vi "GameInit.vi"(8 "error in":errorcluster) -> (0 "error out":errorcluster, 3 "InitCluster":T1)   [LabVIEW 2022 SP3]
uses:
  InitCluster.ctl
  CharacterCluster.ctl
  <vilib>/picture/picture.llb/imagedata.ctl
  ShotInitCluster.ctl
  <vilib>/Utility/miscctls.llb/LVPositionTypeDef.ctl
  <vilib>/Utility/miscctls.llb/LVBoundsTypeDef.ctl
  ShotCluster.ctl
  move_dir_ud.ctl
  SelectPictureToRead.ctl
  ShipShootEnum.ctl
  <vilib>/Utility/config.llb/Read Key (U32).vi
  <vilib>/Utility/config.llb/Read Key (I32).vi
  <vilib>/Utility/config.llb/NI_LVConfig.lvlib
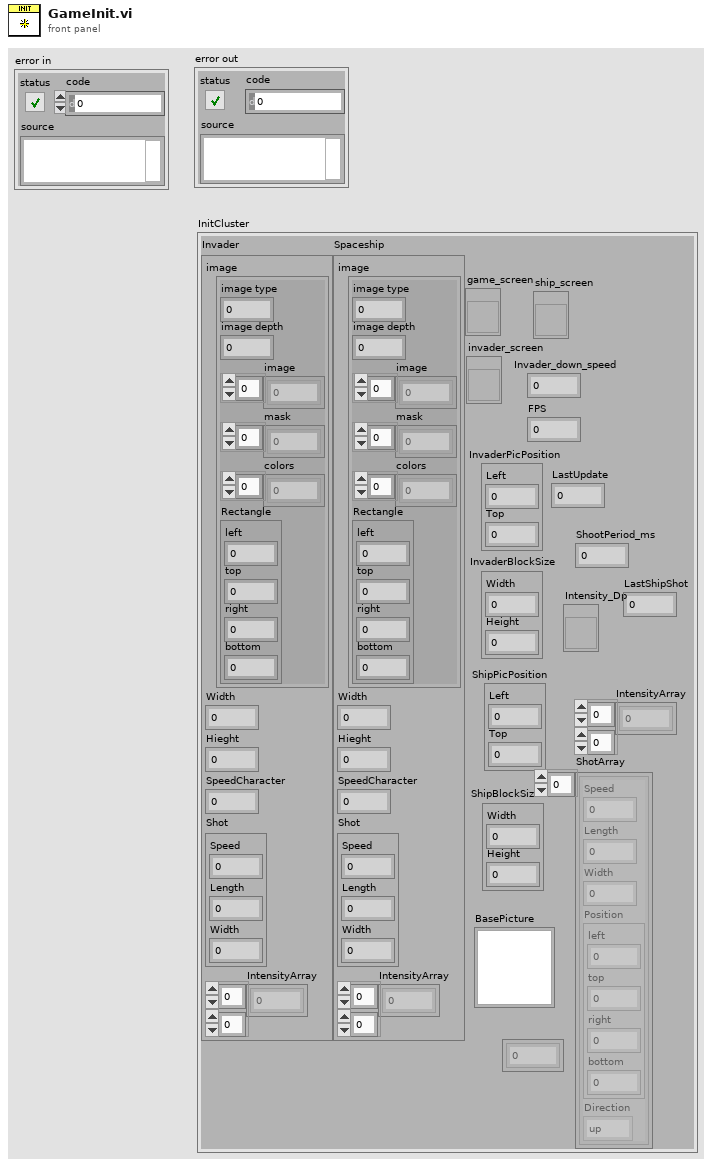
[diagram p1: front panel]
types:
  T1 = typedef "InitCluster.ctl" = cluster{"Invader":T2, "Spaceship":T2, "game_screen":refnum<vi>, "BasePicture":picture, "invader_screen":refnum<vi>, "InvaderPicPosition":T5, "Invader_down_speed":i16, "FPS":u16, "InvaderBlockSize":T6, "ship_screen":refnum<vi>, "ShipBlockSize":T6, "ShipPicPosition":T5, "LastUpdate":u32, "Intensity_Dp":refnum<vi>, "IntensityArray":u8[][], "ShotArray":T7[], "InvaderShotTimeArray":u32[], "ShootPeriod_ms":i32, "LastShipShot":u32}
  T2 = typedef "CharacterCluster.ctl" = cluster{"image":T3, "Width":u32, "Hieght":u32, "SpeedCharacter":u32, "Shot":T4, "IntensityArray":u8[][]}
  T3 = typedef "imagedata.ctl" = cluster{"image type":i32, "image depth":i32, "image":u8[], "mask":u8[], "colors":u32[], "Rectangle":cluster{"left":i16, "top":i16, "right":i16, "bottom":i16}}
  T4 = typedef "ShotInitCluster.ctl" = cluster{"Speed":u32, "Length":u32, "Width":u32}
  T5 = typedef "LVPositionTypeDef.ctl" = cluster{"Left":i32, "Top":i32}
  T6 = typedef "LVBoundsTypeDef.ctl" = cluster{"Width":u32, "Height":u32}
  T7 = typedef "ShotCluster.ctl" = cluster{"Speed":u32, "Length":u32, "Width":u32, "Position":cluster{"left":i16, "top":i16, "right":i16, "bottom":i16}, "Direction":T8}
  T8 = typedef "move_dir_ud.ctl" = enum16{"up", "down"}
  T9 = typedef "ShipShootEnum.ctl" = enum16{"Init", "Read", "Reset"}
  T10 = typedef "SelectPictureToRead.ctl" = enum16{"invader", "spaceship"}
  T11 = typedef "NI_LVConfig.lvlib/Config Data RefNum.ctl" = refnum<k1>
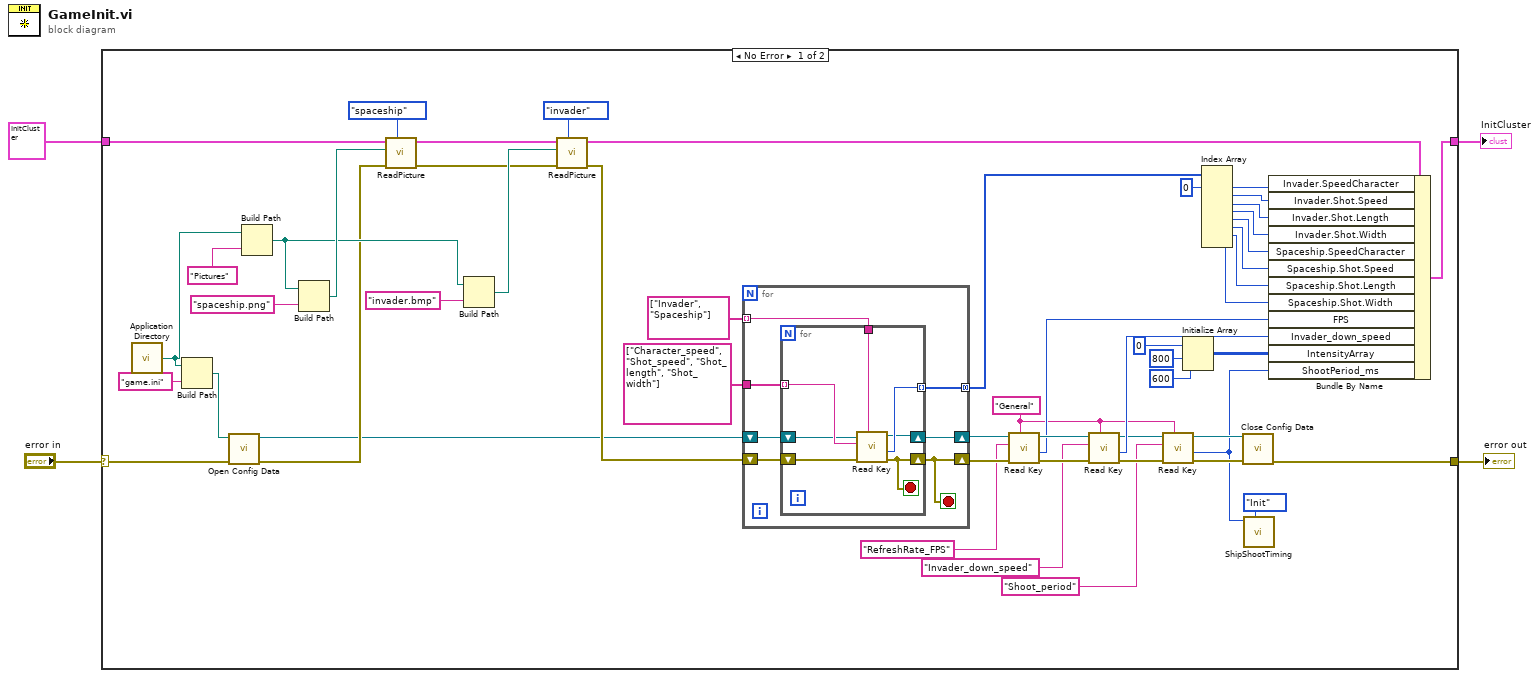
[diagram p0: block diagram]
diagram:
  n1 = case shown="No Error" "error in" {
    selector: "error in" -> [w57 w73]
    tunnel: [w54 w73] -> w3
    tunnel: [w53 w72] -> w2
    tunnel: T1 {"Invader"={"image"={"image type"=0, "image depth"=0, "image"=[], "mask"=[], "colors"=[], "Rectangle"={"left"=0, "top"=0, "right"=0, "bottom"=0}}, "Width"=0, "Hieght"=0, "SpeedCharacter"=0, "Shot"={"Speed"=0, "Length"=0, "Width"=0}, "IntensityArray"=[]}, "Spaceship"={"image"={"image type"=0, "image depth"=0, "image"=[], "mask"=[], "colors"=[], "Rectangle"={"left"=0, "top"=0, "right"=0, "bottom"=0}}, "Width"=0, "Hieght"=0, "SpeedCharacter"=0, "Shot"={"Speed"=0, "Length"=0, "Width"=0}, "IntensityArray"=[]}, "game_screen"=refnum, "BasePicture"=bytes[0], "invader_screen"=refnum, "InvaderPicPosition"={"Left"=0, "Top"=0}, "Invader_down_speed"=0, "FPS"=0, "InvaderBlockSize"={"Width"=0, "Height"=0}, "ship_screen"=refnum, "ShipBlockSize"={"Width"=0, "Height"=0}, "ShipPicPosition"={"Left"=0, "Top"=0}, "LastUpdate"=0, "Intensity_Dp"=refnum, "IntensityArray"=[], "ShotArray"=[], "InvaderShotTimeArray"=[], "ShootPeriod_ms"=0, "LastShipShot"=0} -> [w50 w72]
    frame No Error {
      w18 = "General" ("section")
      n2 = call <vilib>:"Application Directory.vi"() -> ("Application Directory"=w14:path)
      n3 = Build Path(base path=w14, name or relative path="game.ini") -> (appended path=w55:path)
      n4 = call <vilib>:"Open Config Data.vi"("error in (no error)"=w57, "configuration file path"=w55) -> ("error out"=w7:errorcluster, "refnum"=w5:T11)  [unwired: 7 in, 1 out]
      n5 = Build Path(base path=w14, name or relative path="Pictures") -> (appended path=w9:path)
      n6 = Build Path(base path=w9, name or relative path="spaceship.png") -> (appended path=w12:path)
      n7 = call "ReadPicture.vi"("PictureToRead"=SelectPictureToRead."spaceship", "error in"=w7, "path to PNG file"=w12, "InitCluster_IN"=w50) -> ("error out"=w6:errorcluster, "InitCluster_OUT"=w49:T1)  [unwired: 6 in]
      n8 = Build Path(base path=w9, name or relative path="invader.bmp") -> (appended path=w8:path)
      n9 = call "ReadPicture.vi"("PictureToRead"=SelectPictureToRead."invader", "error in"=w6, "path to PNG file"=w8, "InitCluster_IN"=w49) -> ("error out"=w47:errorcluster, "InitCluster_OUT"=w45:T1)  [unwired: 6 in]
      n10 = for {
        tunnel: string[] ["Invader", "Spaceship"] -> [w63] mode=indexing
        tunnel: string[] ["Character_speed", "Shot_speed", "Shot_length", "Shot_width"] -> [w62]
        shift-right: [w58] -> w34
        shift-left: w5 -> [w61]
        shift-right: [w60] -> w33
        shift-left: w47 -> [w64]
        tunnel: [w59] -> w44 mode=concatenating
        stop <- w60 stop-if-true
        n11 = for {
          shift-right: [w65] -> w60
          shift-left: w64 -> [w71]
          tunnel: w63 -> [w70]
          tunnel: w62 -> [w69] mode=indexing
          tunnel: [w68] -> w59 mode=indexing
          shift-right: [w66] -> w58
          shift-left: w61 -> [w67]
          stop <- w65 stop-if-true
          n12 = call-poly <vilib>:"Read Key.vi"("section"=w70, "error in (no error)"=w71, "key"=w69, "refnum"=w67) -> ("error out"=w65:errorcluster, "value"=w68:u32, "refnum out"=w66:T11)  [unwired: 4 in, 1 out]
        }
      }
      n13 = call-poly <vilib>:"Read Key.vi"("section"=w18, "error in (no error)"=w33, "key"="RefreshRate_FPS", "refnum"=w34) -> ("error out"=w31:errorcluster, "value"=w28:i32, "refnum out"=w32:T11)  [unwired: 4 in, 1 out]
      n14 = call-poly <vilib>:"Read Key.vi"("section"=w18, "error in (no error)"=w31, "key"="Invader_down_speed", "refnum"=w32) -> ("error out"=w21:errorcluster, "value"=w23:i32, "refnum out"=w22:T11)  [unwired: 4 in, 1 out]
      n15 = call-poly <vilib>:"Read Key.vi"("section"=w18, "error in (no error)"=w21, "key"="Shoot_period", "refnum"=w22) -> ("error out"=w20:errorcluster, "value"=w15:i32, "refnum out"=w19:T11)  [unwired: 4 in, 1 out]
      n16 = Initialize Array(u8 0, 800 ("dimension size"), 600 ("dimension size")) -> (w24:u8[][])
      n17 = Index Array(array=w44, index #1=0 ("index")) -> (element #1=w43:u32, element #2=w41:u32, element #3=w40:u32, element #4=w39:u32, element #5=w38:u32, element #6=w37:u32, element #7=w36:u32, element #8=w35:u32)  [unwired: 7 in]
      n18 = call <vilib>:"Close Config Data.vi"("error in (no error)"=w20, "refnum"=w19) -> ("error out"=w54:errorcluster)  [unwired: 8 in, 1 out]
      n19 = call "ShipShootTiming.vi"("Selector"=ShipShootEnum."Init", "ShootEnergy"=w15) -> ()  [unwired: 8 in, 2 out]
      n20 = Bundle By Name(cluster=w45, "Invader.SpeedCharacter"=w43, "Invader.Shot.Speed"=w41, "Invader.Shot.Length"=w40, "Invader.Shot.Width"=w39, "Spaceship.SpeedCharacter"=w38, "Spaceship.Shot.Speed"=w37, "Spaceship.Shot.Length"=w36, "Spaceship.Shot.Width"=w35, "FPS"=w28, "Invader_down_speed"=w23, "IntensityArray"=w24, "ShootPeriod_ms"=w15) -> (w53:T1)
    }
    frame Error {
    }
  }
  "error out" <- w3
  "InitCluster" <- w2
